vi "Get settings chain.vi"(8 "error in (no error)":errorcluster, 11 "Example Class A in":refnum<class "ExampleClassA.lvclass">) -> (0 "error out":errorcluster, 1 "class name":string[](array[string]), 2 "settings":variant[](array[variant]), 3 "Example Class A out":refnum<class "ExampleClassA.lvclass">)   [LabVIEW 2012, in "ExampleClassA.lvclass"]
doc: "Returns an array of variants containing the settings clusters of each class in the inheritance chain (lowest child class first), together with an array of all class names in the inheritance chain."
uses:
  ExampleClassA.lvclass
  <vilib>/Distrio/Murmex/Murmex/Murmex.lvclass
  ExampleClassA.lvclass/ExampleClassA.ctl
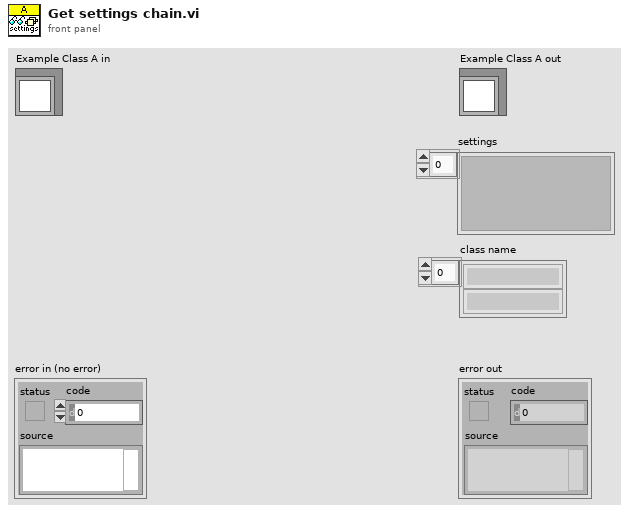
[diagram p1: front panel]
types:
  T1 = typedef "ExampleClassA.lvclass/Settings cluster.ctl" = cluster{"period?":dbl[unit], "number of blocks":i32, "number of channels":i32}
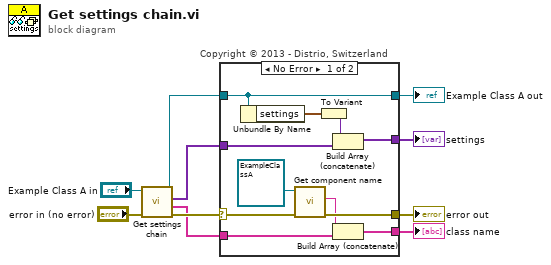
[diagram p0: block diagram]
diagram:
  n1 = call-parent "Get settings chain.vi"("error in (no error)"="error in (no error)", "MurmexBase in"="Example Class A in") -> ("error out"=w8:errorcluster, "class name"=w6:string[], "settings"=w7:variant[], "MurmexBase out"=w1:refnum<class "ExampleClassA.lvclass">)  [unwired: 6 in]
  n2 = case "Copyright © 2013 - Distrio, Switzerland" shown="No Error" w8 {
    selector: w8 -> [w20 w23]
    tunnel: [w21 w23] -> w4
    tunnel: [w18 _] -> w5
    tunnel: [w17 _] -> w2
    tunnel: [w12 w22] -> w3
    tunnel: w7 -> [w15 _]
    tunnel: w6 -> [w16 _]
    tunnel: w1 -> [w12 w22]
    frame No Error {
      n3 = Unbundle By Name(w12) -> ("settings"=w13:T1)
      n4 = call <vilib>:"Get component name.vi"("error in (no error)"=w20, "Murmex in"=refnum<class "ExampleClassA.lvclass"> refnum ("ExampleClassA")) -> ("error out"=w21:errorcluster, "component name"=w19:string)  [unwired: 7 in, 1 out]
      n5 = To Variant(anything=w13) -> (Variant=w14:variant)
      n6 = Build Array (concatenate)(w14, w15) -> (w17:variant[])
      n7 = Build Array (concatenate)(w19, w16) -> (w18:string[])
    }
    frame Error {
    }
  }
  "error out" <- w4
  "Example Class A out" <- w3
  "settings" <- w2
  "class name" <- w5
